vi "G#Debugger_DisconnectFromTypeDef.vi"(0 "Ctl Refnum":refnum<vi>, 5 "error in (no error)":errorcluster) -> (19 "error out":errorcluster)   [LabVIEW 2020, in "G#Debugger.lvlib"]
uses:
  <vilib>/addons/_AddQ/G#Debugger/G#Debugger.lvlib
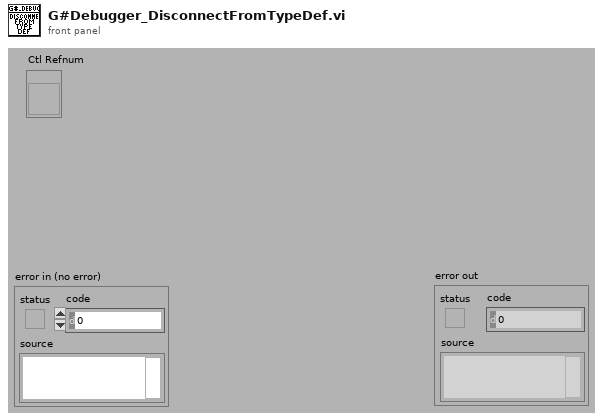
[diagram p1: front panel]
types:
  T1 = enum32{"not a typedef", "typedef", "strict typedef", "class private data"}
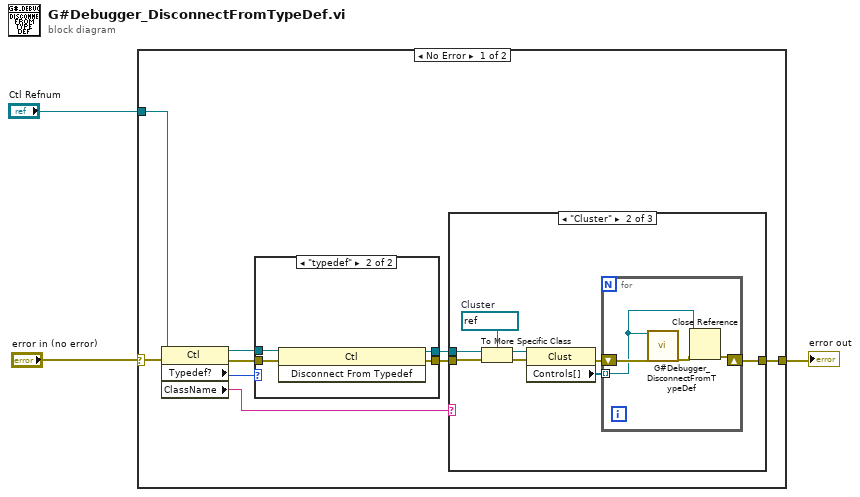
[diagram p0: block diagram]
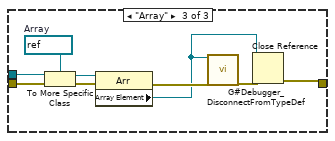
[diagram p3: hidden frame]
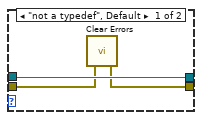
[diagram p4: hidden frame]
diagram:
  n1 = case shown="No Error" "error in (no error)" {
    selector: "error in (no error)" -> [w4 w42]
    tunnel: "Ctl Refnum" -> [w6 _]
    tunnel: [w5 w42] -> w2
    frame No Error {
      n2 = property class="Ctl"(reference=w6, error in=w4) -> (reference out=w11:refnum<vi>, error out=w12:errorcluster, "Typedef?"=w10:T1, "ClassName"=w9:string)
      n3 = case shown="\"typedef\"" w10 {
        tunnel: w12 -> [w36 w41]
        tunnel: w11 -> [w37 w40]
        tunnel: [w35 w39] -> w8
        tunnel: [w37 w38] -> w7
        frame "not a typedef", Default {
          n4 = call <vilib>:"Clear Errors.vi"("error in (no error)"=w36) -> ("error out"=w35:errorcluster)  [unwired: 5 in, 1 out]
        }
        frame "typedef" {
          n5 = invoke class="Ctl" method="Disconnect From Typedef"(reference=w40, error in=w41) -> (reference out=w38:refnum<vi>, error out=w39:errorcluster)  [unwired: 1 in, 1 out]
        }
      }
      n6 = case shown="\"Cluster\"" w9 {
        tunnel: w8 -> [w13 w21 w31]
        tunnel: w7 -> [_ w20 w30]
        tunnel: [w13 w14 w29] -> w5
        frame Default {
        }
        frame "Cluster" {
          w19 = refnum<vi> refnum  # Cluster
          n7 = To More Specific Class(target class=w19, reference=w20, error in=w21) -> (specific class reference=w18:refnum<vi>, error out=w17:errorcluster)
          n8 = property class="Clust"(reference=w18, error in=w17) -> (error out=w16:errorcluster, "Controls[]"=w15:refnum<vi>[])  [unwired: 1 out]
          n9 = for {
            shift-right: [w25] -> w14
            shift-left: w16 -> [w24]
            tunnel: w15 -> [w22] mode=indexing
            n10 = call <vilib>:"G#Debugger_DisconnectFromTypeDef.vi"("Ctl Refnum"=w22, "error in (no error)"=w24) -> ("error out"=w23:errorcluster)  [unwired: 17 in]
            n11 = Close Reference(reference=w22, error in (no error)=w23) -> (error out=w25:errorcluster)
          }
        }
        frame "Array" {
          w34 = refnum<vi> refnum  # Array
          n12 = To More Specific Class(target class=w34, reference=w30, error in=w31) -> (specific class reference=w33:refnum<vi>, error out=w32:errorcluster)
          n13 = property class="Arr"(reference=w33, error in=w32) -> (error out=w28:errorcluster, "Array Element"=w26:refnum<vi>)  [unwired: 1 out]
          n14 = call <vilib>:"G#Debugger_DisconnectFromTypeDef.vi"("Ctl Refnum"=w26, "error in (no error)"=w28) -> ("error out"=w27:errorcluster)  [unwired: 17 in]
          n15 = Close Reference(reference=w26, error in (no error)=w27) -> (error out=w29:errorcluster)
        }
      }
    }
    frame Error {
    }
  }
  "error out" <- w2
